vi "EPM_Power (Single Phase).vi"(8 "error in (no error)":errorcluster, 10 "Current":waveform(dbl), 11 "Voltage":waveform(dbl)) -> (0 "error out":errorcluster, 1 "Irms":dbl format="%0.2f", 2 "Vrms":dbl format="%0.2f", 3 "Power":T1)   [LabVIEW 2019, in "Main.lvclass"]
doc: "Developed by Kevin Thompson\nkevin@thompsonengineering.net\n\nCopyright 2020\nThompson Engineering, LLC\nThis VI calculates the power in a single phase AC or DC signal. The integration time for the measurement is equal to the duration of the time domain waveform. For the best measurement accuracy on the AC signal, input time domain data of at least 10 cycles."
uses:
  Main.lvclass
  <vilib>/Analysis/baseanly.llb/Mean (DBL).vi
  <vilib>/Analysis/NI_AALPro.lvlib
  <vilib>/Analysis/NI_AALBase.lvlib
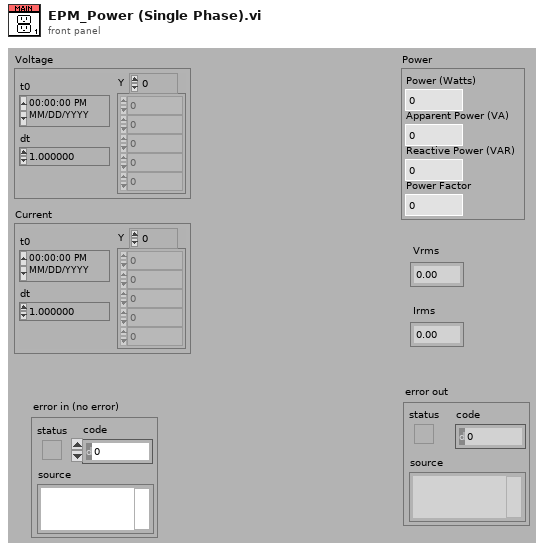
[diagram p1: front panel]
types:
  T1 = cluster{"Power (Watts)":dbl, "Apparent Power (VA)":dbl, "Reactive Power (VAR)":dbl, "Power Factor":dbl}
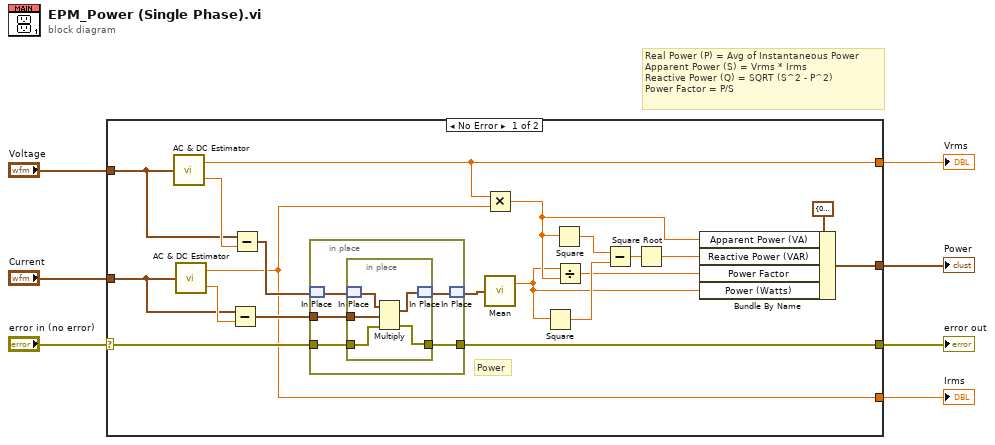
[diagram p0: block diagram]
diagram:
  # "Real Power (P) = Avg of Instantaneous Power\nApparent Power (S) = Vrms * Irms\nReactive Power (Q) = SQRT (S^2 - P^2)\nPower Factor = P/S"
  n1 = case shown="No Error" "error in (no error)" {
    selector: "error in (no error)" -> [w27 w38]
    tunnel: "Voltage" -> [w17 _]
    tunnel: "Current" -> [w14 _]
    tunnel: [w26 w38] -> w6
    tunnel: [w12 _] -> w3
    tunnel: [w10 _] -> w2
    tunnel: [w9 _] -> w1
    frame No Error {
      # "Power"
      n2 = call <vilib>:"AC & DC Estimator.vi"("Signal (V)"=w17) -> ("AC estimate (Vrms)"=w10:dbl, "DC estimate (V)"=w18:dbl)
      n3 = call <vilib>:"AC & DC Estimator.vi"("Signal (V)"=w14) -> ("AC estimate (Vrms)"=w9:dbl, "DC estimate (V)"=w15:dbl)
      n4 = Subtract(x=w14, y=w15) -> (x-y=w13:waveform(dbl))
      n5 = Subtract(x=w17, y=w18) -> (x-y=w16:waveform(dbl))
      n6 = in-place {
        in-place-border: w13 -> [w32]
        in-place-border: w27 -> [w31]
        in-place-border: [w30] -> w26
        n7 = in-place-match #1(w16) -> (w29:waveform(dbl))
        n8 = in-place {
          in-place-border: w32 -> [w37]
          in-place-border: w31 -> [w36]
          in-place-border: [w35] -> w30
          n9 = in-place-match #2(w29) -> (w34:waveform(dbl))
          n10 = Multiply(1:w37, 2:w34, 4:w36) -> (0:w33:waveform(dbl), 3:w35:errorcluster)
          n11 = in-place-match #2(w33) -> (w28:waveform(dbl))
        }
        n12 = in-place-match #1(w28) -> (w19:waveform(dbl))
      }
      n13 = Multiply(x=w10, y=w9) -> (x*y=w25:dbl)
      n14 = call-poly <vilib>:"Mean.vi"("X"=w19) -> ("mean"=w8:dbl)  [unwired: 1 out]
      n15 = Square(x=w8) -> (x^2=w24:dbl)
      n16 = Square(x=w25) -> (x^2=w23:dbl)
      n17 = Divide(x=w8, y=w25) -> (x/y=w20:dbl)
      n18 = Subtract(x=w23, y=w24) -> (x-y=w22:dbl)
      n19 = Square Root(x=w22) -> (sqrt(x)=w21:dbl)
      n20 = Bundle By Name(cluster=T1 {"Power (Watts)"=0.0, "Apparent Power (VA)"=0.0, "Reactive Power (VAR)"=0.0, "Power Factor"=0.0} ("Total Power Data"), "Apparent Power (VA)"=w25, "Reactive Power (VAR)"=w21, "Power Factor"=w20, "Power (Watts)"=w8) -> (w12:T1)
    }
    frame Error {
    }
  }
  "error out" <- w6
  "Power" <- w3
  "Vrms" <- w2
  "Irms" <- w1
